vi "Pi-Drive - Norm 2 Values (SubVI).vi"(9 "Max Value":dbl=1.0, 10 "Value 2":dbl, 11 "Value 1":dbl) -> (2 "Output Value 2":dbl, 3 "Output Value 1":dbl)   [LabVIEW 2019]
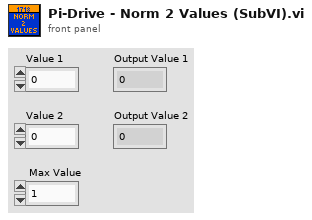
[diagram p1: front panel]
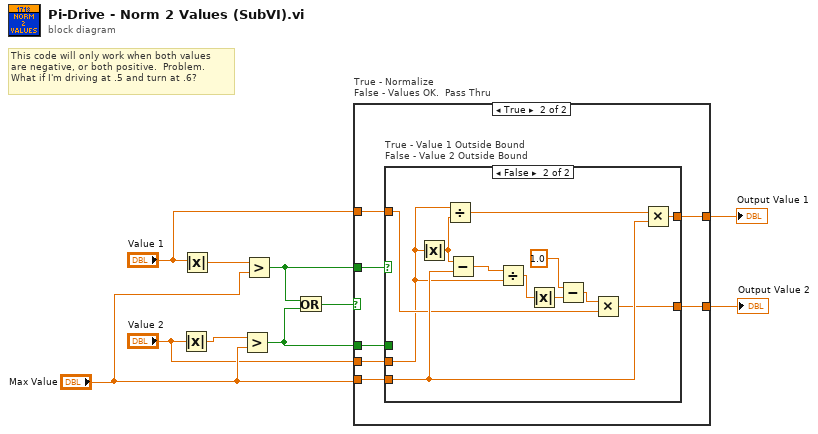
[diagram p0: block diagram]
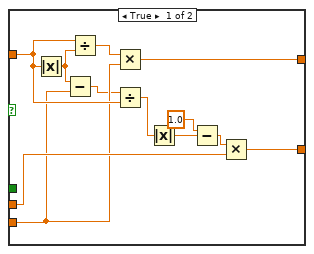
[diagram p3: hidden frame]
diagram:
  # "This code will only work when both values\nare negative, or both positive.  Problem.\nWhat if I'm driving at .5 and turn at .6?"
  n1 = Absolute Value(x="Value 2") -> (abs(x)=w5:dbl)
  n2 = Absolute Value(x="Value 1") -> (abs(x)=w4:dbl)
  n3 = Greater?(x=w5, y="Max Value") -> (0:w1:bool)
  n4 = Greater?(x=w4, y="Max Value") -> (0:w2:bool)
  n5 = Or(x=w2, y=w1) -> (x .or. y?=w3:bool)
  n6 = case "True - Normalize\nFalse - Values OK.  Pass Thru" shown="True" w3 {
    tunnel: [w12 w14] -> w6
    tunnel: "Value 1" -> [w12 w19]
    tunnel: [w11 w13] -> w7
    tunnel: "Value 2" -> [w11 w18]
    tunnel: "Max Value" -> [_ w17]
    tunnel: w2 -> [_ w16]
    tunnel: w1 -> [_ w15]
    frame False {
    }
    frame True {
      n7 = case "True - Value 1 Outside Bound\nFalse - Value 2 Outside Bound" shown="False" w16 {
        tunnel: w19 -> [w31 w35]
        tunnel: w18 -> [w30 w34]
        tunnel: w17 -> [w29 w43]
        tunnel: w15 -> [_ _]
        tunnel: [w28 w32] -> w14
        tunnel: [w27 w33] -> w13
        frame True {
          n8 = Absolute Value(x=w31) -> (abs(x)=w24:dbl)
          n9 = Subtract(x=w24, y=w29) -> (x-y=w26:dbl)
          n10 = Divide(x=w31, y=w24) -> (x/y=w23:dbl)
          n11 = Multiply(x=w23, y=w29) -> (x*y=w28:dbl)
          n12 = Divide(x=w26, y=w31) -> (x/y=w25:dbl)
          n13 = Absolute Value(x=w25) -> (abs(x)=w22:dbl)
          n14 = Subtract(x=1.0, y=w22) -> (x-y=w20:dbl)
          n15 = Multiply(x=w20, y=w30) -> (x*y=w27:dbl)
        }
        frame False {
          n16 = Absolute Value(x=w34) -> (abs(x)=w40:dbl)
          n17 = Divide(x=w34, y=w40) -> (x/y=w39:dbl)
          n18 = Subtract(x=w40, y=w43) -> (x-y=w42:dbl)
          n19 = Divide(x=w42, y=w34) -> (x/y=w41:dbl)
          n20 = Absolute Value(x=w41) -> (abs(x)=w38:dbl)
          n21 = Subtract(x=1.0, y=w38) -> (x-y=w36:dbl)
          n22 = Multiply(x=w36, y=w35) -> (x*y=w32:dbl)
          n23 = Multiply(x=w39, y=w43) -> (x*y=w33:dbl)
        }
      }
    }
  }
  "Output Value 2" <- w7
  "Output Value 1" <- w6
